vi "Conductus Write Set Point.vi"(1 "Setpoint":dbl=4.21 min=0.0 max=1000.0 step=0.001 format="%.3f", 2 "Instrument Address":refnum<visa-resource-name>) -> ()   [LabVIEW 2024]
doc: "Changes the setpoint for sensor #1 on a conductus LTC20 Temperature controller.\nScott Hannahs, NHMFL-FSU, Feb 1996"
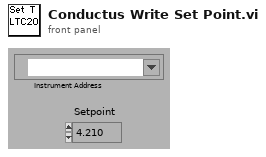
[diagram p1: front panel]
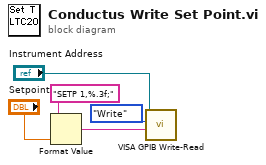
[diagram p0: block diagram]
diagram:
  n1 = Format Value(format string="SETP 1,%.3f;", value (0)="Setpoint") -> (output string=w3:string)  [unwired: 1 in]
  n2 = call "VISA GPIB Write-Read.vi"("Command"=w3, "Action"=enum16{"Write", "Read", "Write & Read"}."Write", "VISA resource name"="Instrument Address") -> ()  [unwired: 5 in, 4 out]
